vi "Alpha4.0.2.vi"() -> ()   [LabVIEW 2011]
uses:
  <vilib>/vision/NI_Vision_Development_Module.lvlib
panel:
  out "Disabled":T1(ring)
  in  "Manual Threshold":T2(array[cluster]) {"Lower Limit" scale=0.0..255.0; "Upper Limit" scale=0.0..255.0; "Replace Value" format="%.2f"}
  in  "Look for...":u16(ring) items=["Bright Objects", "Dark Objects"]
  in  "Local Threshold Method":u16(ring) items=["Niblack", "Background Correction"]
  in  "Threshold selectoin":bool
  out "Image Enhanced":T3(plugin-control)
  in  "Gamma":sgl(slide)=2.14 scale=0.0..10.0
  in  "Contrast":u8(slide)=60 scale=0.0..255.0
  in  "Brightness":u8(slide)=118 scale=0.0..255.0
  in  "Basic Morphology Operatoin":T4(ring)
  out "Threshold":T3(plugin-control)
  in  "Stop":bool
  in  "Browse":bool
  out "Original Image":T3(plugin-control)
  out "Path to Image":path
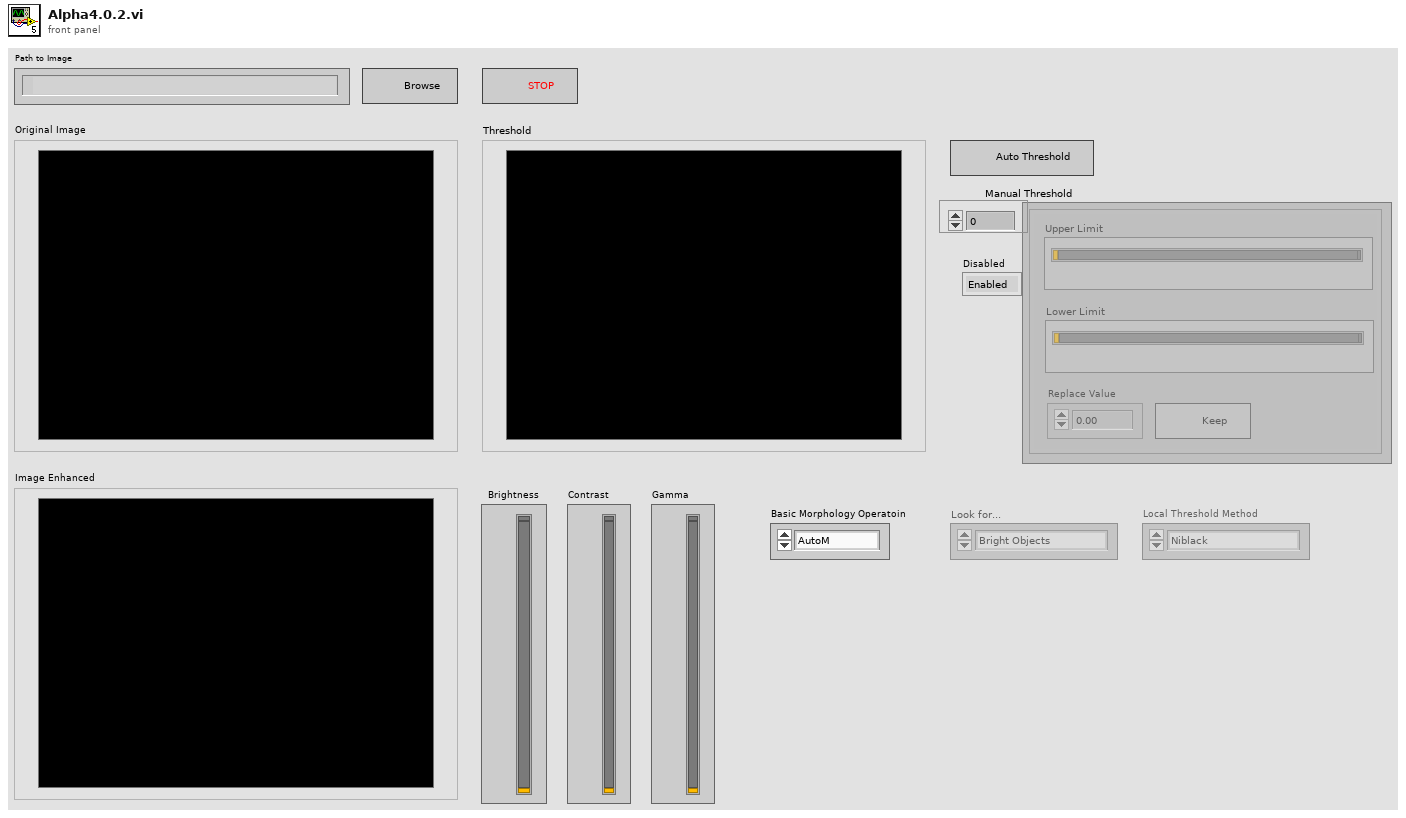
[diagram p1: front panel]
types:
  T1 = enum8{"Enabled", "Disabled", "Disabled and Grayed Out"}
  T2 = cluster{"Upper Limit":sgl, "Lower Limit":sgl, "Replace Value":sgl, "Keep/Replace Value (Replace)":bool}[]
  T3 = typedef "IMAQ Image.ctl" = refnum<image>
  T4 = enum16{"AutoM", "Close", "Dilate", "Erode", "Gradient", "Gradient out", "Gradient in", "Hit miss", "Open", "PClose", "POpen", "Thick", "Thin"}
  T5 = typedef "Image Type" = u32
  T6 = cluster{"Brightness":u8, "Contrast":u8, "Gamma":sgl}
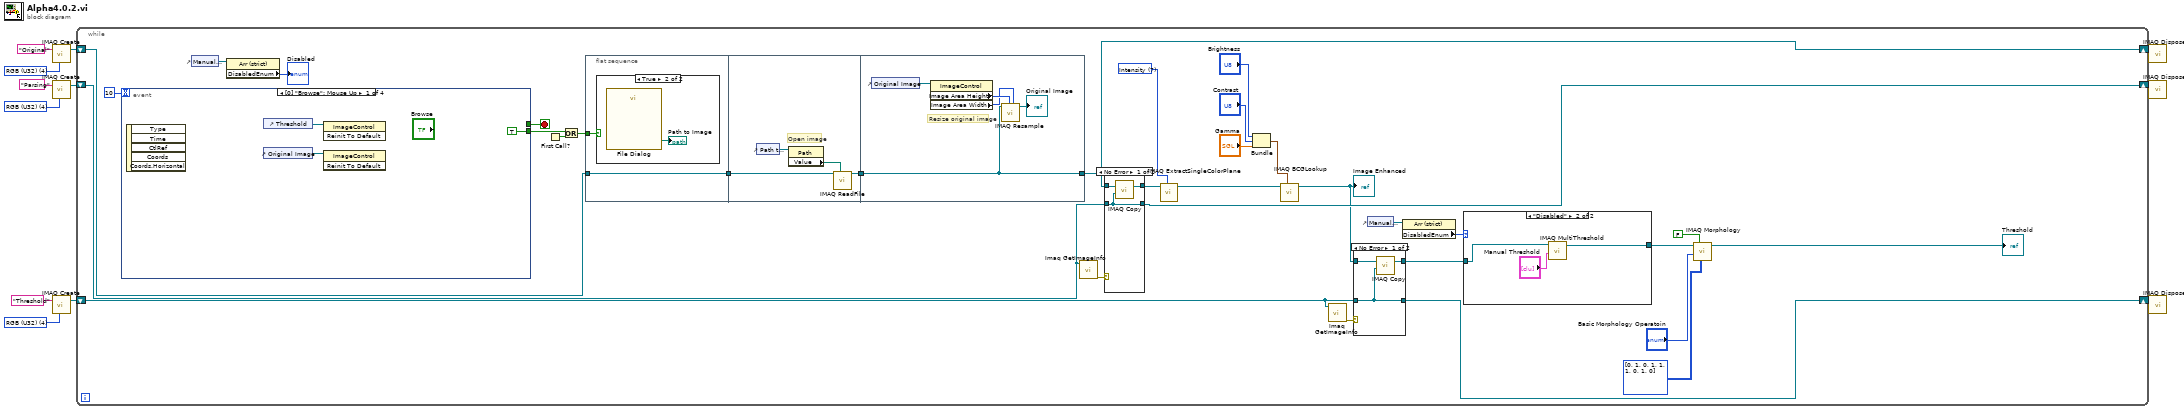
[diagram p0: block diagram]
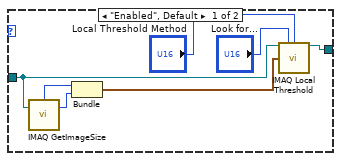
[diagram p2: hidden frame]
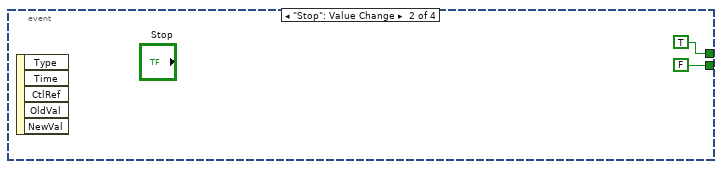
[diagram p6: hidden frame]
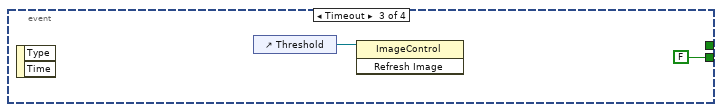
[diagram p7: hidden frame]
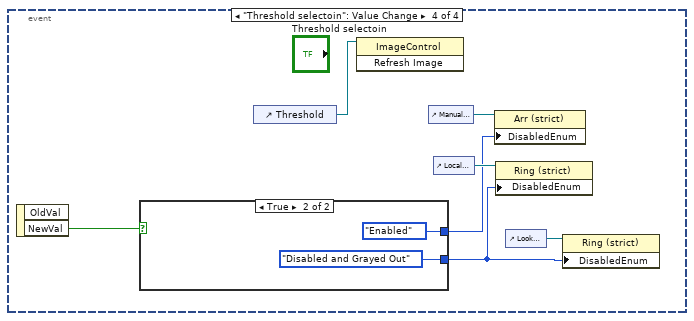
[diagram p8: hidden frame]
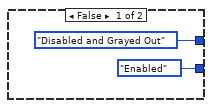
[diagram p9: hidden frame]
diagram:
  w3 = T5 4 items=["Grayscale (U8)", "Grayscale (I16)", "Grayscale (SGL)", "Complex (CSG)", "RGB (U32)", "HSL (U32)", "RGB (U64)", "Grayscale (U16)"] ("Image Type")
  w5 = T5 4 items=["Grayscale (U8)", "Grayscale (I16)", "Grayscale (SGL)", "Complex (CSG)", "RGB (U32)", "HSL (U32)", "RGB (U64)", "Grayscale (U16)"] ("Image Type")
  w8 = T5 4 items=["Grayscale (U8)", "Grayscale (I16)", "Grayscale (SGL)", "Complex (CSG)", "RGB (U32)", "HSL (U32)", "RGB (U64)", "Grayscale (U16)"] ("Image Type")
  n1 = call "IMAQ Create"("Image Name"="Original", "Image Type"=w8) -> ("New Image"=w11:T3)  [unwired: 3 in, 1 out]
  n2 = call "IMAQ Create"("Image Name"="Parsing", "Image Type"=w5) -> ("New Image"=w9:T3)  [unwired: 3 in, 1 out]
  n3 = call "IMAQ Create"("Image Name"="Threshold", "Image Type"=w3) -> ("New Image"=w2:T3)  [unwired: 3 in, 1 out]
  n4 = while {
    shift-right: [w42] -> w7
    shift-left: w11 -> [w37]
    shift-right: [w24] -> w6
    shift-left: w9 -> [w41]
    shift-right: [w21] -> w1
    shift-left: w2 -> [w22]
    stop <- w43 stop-if-true
    w28 = 7 items=["Red", "Green", "Blue", "Hue", "Saturation", "Luminance", "Value", "Intensity"] ("Color Plane")
    n5 = event shown="[0] \"Browse\": Mouse Up" {
      selector: _ -> [_ _ _ _]
      dyn-events: _ -> [_ _ _ _]
      timeout: 10 -> [_ _ _ _]
      tunnel: [_ TRUE _ _] -> w43
      tunnel: [TRUE FALSE FALSE _] -> w40
      event "Browse": Mouse Up {
        n6 = event-data() -> ()  [unwired: 1 in, 5 out]
        n7 = control-ref of="Threshold"() -> (w80:refnum<vi>)
        n8 = control-ref of="Original Image"() -> (w79:refnum<vi>)
        n9 = invoke class="ImageControl" method="Reinit To Default"(reference=w80) -> ()  [unwired: 2 in, 3 out]
        n10 = invoke class="ImageControl" method="Reinit To Default"(reference=w79) -> ()  [unwired: 2 in, 3 out]
      }
      event "Stop": Value Change {
        n11 = event-data() -> ()  [unwired: 1 in, 5 out]
      }
      event Timeout {
        n12 = event-data() -> ()  [unwired: 1 in, 2 out]
        n13 = control-ref of="Threshold"() -> (w84:refnum<vi>)
        n14 = invoke class="ImageControl" method="Refresh Image"(reference=w84) -> ()  [unwired: 2 in, 3 out]
      }
      event "Threshold selectoin": Value Change {
        n15 = event-data() -> ("NewVal"=w91:bool)  [unwired: 1 in, 1 out]
        n16 = case shown="True" w91 {
          tunnel: [T1."Disabled and Grayed Out" ("Disabled") T1."Enabled" ("Disabled")] -> w85
          tunnel: [T1."Enabled" ("Disabled") T1."Disabled and Grayed Out" ("Disabled")] -> w88
          frame False {
          }
          frame True {
          }
        }
        n17 = control-ref of="Threshold"() -> (w87:refnum<vi>)
        n18 = invoke class="ImageControl" method="Refresh Image"(reference=w87) -> ()  [unwired: 2 in, 3 out]
        n19 = control-ref of="Manual Threshold"() -> (w86:refnum<vi>)
        n20 = control-ref of="Local Threshold Method"() -> (w89:refnum<vi>)
        n21 = property class="Arr (strict)"(reference=w86, "DisabledEnum"=w85) -> ()  [unwired: 1 in, 2 out]
        n22 = property class="Ring (strict)"(reference=w89, "DisabledEnum"=w88) -> ()  [unwired: 1 in, 2 out]
        n23 = control-ref of="Look for..."() -> (w90:refnum<vi>)
        n24 = property class="Ring (strict)"(reference=w90, "DisabledEnum"=w88) -> ()  [unwired: 1 in, 2 out]
      }
    }
    n25 = control-ref of="Manual Threshold"() -> (w15:refnum<vi>)
    n26 = property class="Arr (strict)"(reference=w15) -> ("DisabledEnum"=→"Disabled":T1)  [unwired: 1 in, 2 out]
    n27 = First Call?() -> (First Call?: T/F=w39:bool)
    n28 = Or(x=w40, y=w39) -> (x .or. y?=w38:bool)
    n29 = flat-sequence {
      tunnel: w38 -> [w67]
      tunnel: w37 -> [w66]
      tunnel: [w66] -> w36
      tunnel: [w72] -> w45
      tunnel: w36 -> [w69]
      tunnel: w45 -> [w73]
      tunnel: [w73] -> w42
      frame #0 {
        n30 = case shown="True" w67 {
          frame False {
          }
          frame True {
            n31 = call "File Dialog"() -> ("selected path"=→"Path to Image":path)  [unwired: 12 in, 3 out]
          }
        }
      }
      frame #1 {
        # "Open image"
        n32 = control-ref of="Path to Image"() -> (w71:refnum<vi>)
        n33 = property class="Path"(reference=w71) -> ("Value"=w70:path)  [unwired: 1 in, 2 out]
        n34 = call "IMAQ ReadFile"("File Path"=w70, "Image"=w69) -> ("Image Out"=w72:T3)  [unwired: 5 in, 4 out]
      }
      frame #2 {
        # "Resize original image"
        n35 = control-ref of="Original Image"() -> (w77:refnum<vi>)
        n36 = property class="ImageControl"(reference=w77) -> ("Image Area Height"=w76:u32, "Image Area Width"=w75:u32)  [unwired: 1 in, 2 out]
        n37 = call "IMAQ Resample"("X Resolution"=w75, "Y Resolution"=w76, "Image Src"=w73) -> ("Image Dst Out"=→"Original Image":T3)  [unwired: 7 in, 1 out]
      }
    }
    n38 = call "Imaq GetImageInfo"("Image"=w41) -> ("error out"=w44:errorcluster)  [unwired: 1 in, 9 out]
    n39 = case shown="No Error" w44 {
      tunnel: w41 -> [w61 w64]
      tunnel: w42 -> [w63 w65]
      tunnel: [w62 w65] -> w25
      tunnel: [w61 w64] -> w24
      frame No Error {
        n40 = call "IMAQ Copy"("Image Dst"=w61, "Image Src"=w63) -> ("Image Dst Out"=w62:T3)  [unwired: 4 in, 1 out]
      }
      frame Error {
      }
    }
    n41 = call "IMAQ ExtractSingleColorPlane"("Color Plane"=w28, "Image Src"=w25) -> ("Image Dst Out"=w29:T3)  [unwired: 2 in, 7 out]
    n42 = Bundle("Brightness"="Brightness", "Contrast"="Contrast", "Gamma"="Gamma") -> (w27:T6)  [unwired: 1 in]
    n43 = call "IMAQ BCGLookup"("Image Src"=w29, "BCG Values"=w27) -> ("Image Dst Out"=w20:T3)  [unwired: 3 in, 3 out]
    "Image Enhanced" <- w20
    n44 = call "Imaq GetImageInfo"("Image"=w22) -> ("error out"=w23:errorcluster)  [unwired: 1 in, 9 out]
    n45 = case shown="No Error" w23 {
      tunnel: w22 -> [w56 w59]
      tunnel: w20 -> [w58 w60]
      tunnel: [w57 w60] -> w18
      tunnel: [w56 w59] -> w21
      frame No Error {
        n46 = call "IMAQ Copy"("Image Dst"=w56, "Image Src"=w58) -> ("Image Dst Out"=w57:T3)  [unwired: 4 in, 1 out]
      }
      frame Error {
      }
    }
    n47 = control-ref of="Manual Threshold"() -> (w17:refnum<vi>)
    n48 = property class="Arr (strict)"(reference=w17) -> ("DisabledEnum"=w16:T1)  [unwired: 1 in, 2 out]
    n49 = case shown="\"Disabled\"" w16 {
      tunnel: [w52 w55] -> w19
      tunnel: w18 -> [w49 w54]
      frame "Enabled", Default {
        n50 = call "IMAQ GetImageSize"("Image"=w49) -> ("Y Resolution"=w51:i32, "X Resolution"=w50:i32)  [unwired: 1 in, 3 out]
        n51 = Bundle("X Resolution"=w50, "Y Resolution"=w51) -> (w48:cluster{"X Resolution":i32, "Y Resolution":i32})  [unwired: 1 out]
        n52 = call "IMAQ Local Threshold"("Image Src"=w49, "Look For (Bright Objects)"="Look for...", "Method (Niblack)"="Local Threshold Method", "Window Size (32x32)"=w48) -> ("Image Dst Out"=w52:T3)  [unwired: 10 in, 1 out]
      }
      frame "Disabled" {
        n53 = call "IMAQ MultiThreshold"("Threshold Data"="Manual Threshold", "Image Src"=w54) -> ("Image Dst Out"=w55:T3)  [unwired: 3 in, 1 out]
      }
    }
    n54 = call "IMAQ Morphology"("Structuring Element"=i32[][] [[0, 1, 0], [1, 1, 1], [0, 1, 0]], "Square/Hexa (Square)"=FALSE, "Operation"="Basic Morphology Operatoin", "Image Src"=w19) -> ("Image Dst Out"=→"Threshold":T3)  [unwired: 3 in, 4 out]
  }
  n55 = call "IMAQ Dispose"("Image"=w7) -> ()  [unwired: 5 in, 1 out]
  n56 = call "IMAQ Dispose"("Image"=w6) -> ()  [unwired: 5 in, 1 out]
  n57 = call "IMAQ Dispose"("Image"=w1) -> ()  [unwired: 5 in, 1 out]
